vi "AODO-Write (AO).vi"(0 "Tasks In":T1[](array[typedef]), 7 "AO Waveforms":dbl[][](array[numeric]), 11 "error in (no error)":errorcluster) -> (4 "Tasks Out":T1[](array[typedef]), 15 "error out":errorcluster)   [LabVIEW 2020]
uses:
  Typedefs/AODO-Task Specification.ctl
  <vilib>/DAQmx/write.llb/DAQmx Write (Analog 2D DBL NChan NSamp).vi
  <vilib>/DAQmx/write.llb/DAQmx Write (Analog 1D DBL 1Chan NSamp).vi
  <vilib>/DAQmx/miscellaneous.llb/DAQmx Fill In Error Info.vi
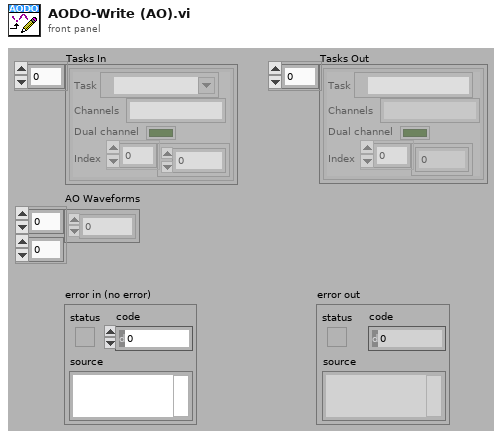
[diagram p1: front panel]
types:
  T1 = typedef "AODO-Task Specification.ctl" = cluster{"Task":refnum<k21>, "Channels":string, "Dual channel":bool, "Index":i32[]}
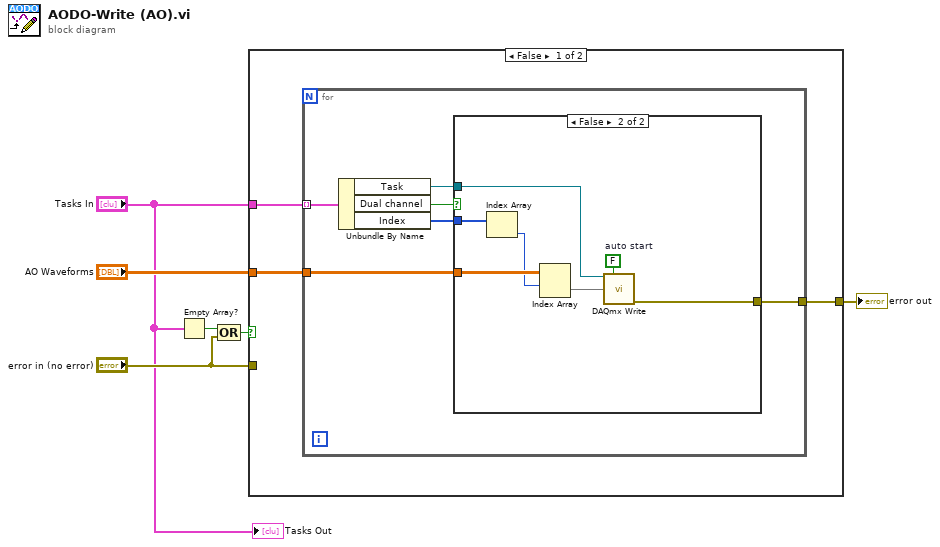
[diagram p0: block diagram]
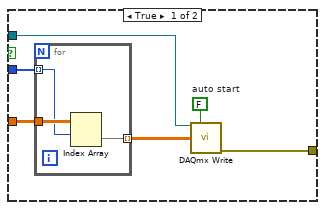
[diagram p2: hidden frame]
diagram:
  n1 = Empty Array?(array="Tasks In") -> (empty?=w2:bool)
  n2 = Compound Arithmetic op=OR(w2, "error in (no error)") -> (w5:bool)
  n3 = case shown="False" w5 {
    tunnel: [w9 w32] -> w6
    tunnel: "error in (no error)" -> [_ w32]
    tunnel: "Tasks In" -> [w8 _]
    tunnel: "AO Waveforms" -> [w7 _]
    frame False {
      n4 = for {
        tunnel: w8 -> [w12] mode=indexing
        tunnel: w7 -> [w14]
        tunnel: [w15] -> w9
        n5 = Unbundle By Name(w12) -> ("Task"=w11:refnum<k21>, "Dual channel"=w13:bool, "Index"=w10:i32[])
        n6 = case shown="False" w13 {
          tunnel: w11 -> [w17 w26]
          tunnel: [w21 w31] -> w15
          tunnel: w14 -> [w20 w30]
          tunnel: w10 -> [w19 w28]
          frame True {
            w18 = FALSE  # auto start
            n7 = for {
              tunnel: w20 -> [w24]
              tunnel: [w22] -> w16 mode=indexing
              tunnel: w19 -> [w23] mode=indexing
              n8 = Index Array(array=w24, index (row)=w23) -> (element=w22:dbl[])  [unwired: 1 in]
            }
            n9 = call-poly <vilib>:"DAQmx Write.vi"("task/channels in"=w17, "auto start"=w18, "data"=w16) -> ("error out"=w21:errorcluster)  [unwired: 10 in, 2 out]
          }
          frame False {
            w29 = FALSE  # auto start
            n10 = Index Array(array=w28) -> (element=w27:i32)  [unwired: 1 in]
            n11 = Index Array(array=w30, index (row)=w27) -> (element=w25:dbl[])  [unwired: 1 in]
            n12 = call-poly <vilib>:"DAQmx Write.vi"("task/channels in"=w26, "auto start"=w29, "data"=w25) -> ("error out"=w31:errorcluster)  [unwired: 10 in, 2 out]
          }
        }
      }
    }
    frame True {
    }
  }
  "error out" <- w6
  "Tasks Out" <- "Tasks In"
